vi "BCG Lookup.vi"() -> ()   [LabVIEW 2014]
doc: "This example shows how to apply a brightness, contrast, and gamma correction lookup table to an image. These transformations are usually applied to an image to improve its quality as required by a particular application."
uses:
  <vilib>/vision/NI_Vision_Development_Module.lvlib
panel:
  in  "Stop Button":bool
  out "Processed Image":T1(plugin-control)
  out "Image Source":T1(plugin-control)
  in  "BCG Values":T2={"Brightness"=171.0, "Contrast"=56.0, "Gamma"=2.0} {"Gamma" min=0.1 max=10 step=0.01 scale=10.0..0.1; "Contrast" min=1 max=89 step=1 scale=30.0..60.0; "Brightness" min=0 max=255 step=1 scale=0.0..255.0}
  # "Overview: Demonstrates how to improve the appearance of an image by changing brightness, contrast and gamma.\nRequirements: NI Vision Development Module\nInstructions: Run the VI."
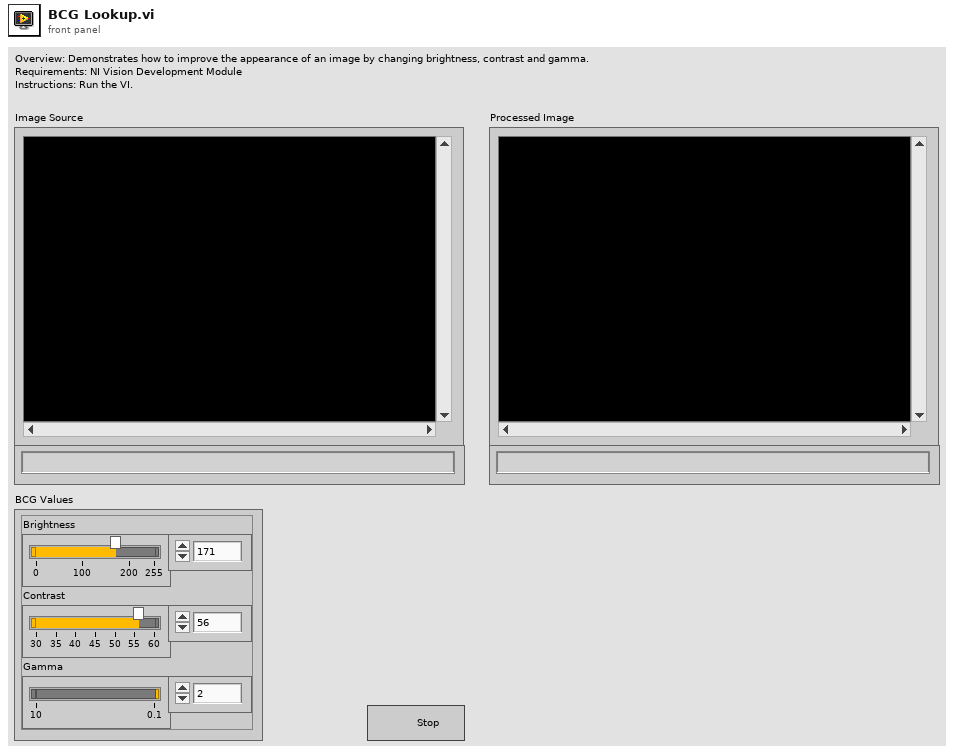
[diagram p1: front panel]
types:
  T1 = typedef "IMAQ Image.ctl" = refnum<image>
  T2 = cluster{"Brightness":sgl, "Contrast":sgl, "Gamma":sgl}
  T3 = typedef "Image Type" = u32
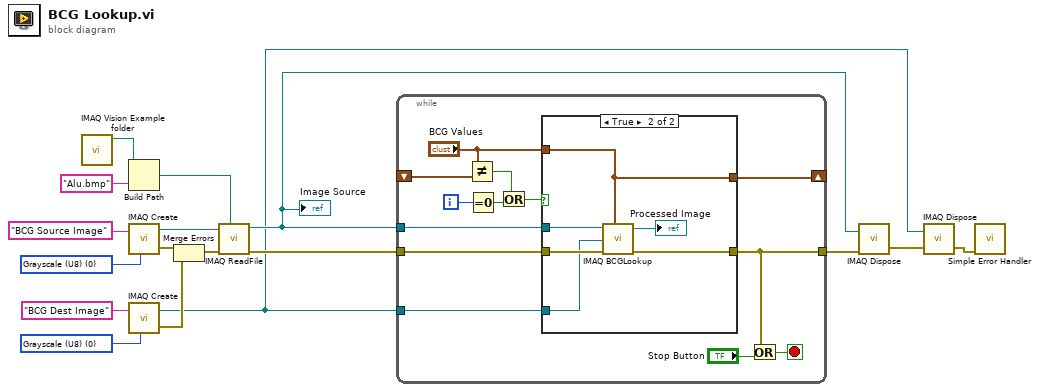
[diagram p0: block diagram]
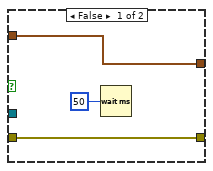
[diagram p2: hidden frame]
diagram:
  w8 = T3 0 items=["Grayscale (U8)", "Grayscale (I16)", "Grayscale (SGL)", "Complex (CSG)", "RGB (U32)", "HSL (U32)", "RGB (U64)", "Grayscale (U16)"] ("Image Type")
  w9 = T3 0 items=["Grayscale (U8)", "Grayscale (I16)", "Grayscale (SGL)", "Complex (CSG)", "RGB (U32)", "HSL (U32)", "RGB (U64)", "Grayscale (U16)"] ("Image Type")
  n1 = call "IMAQ Vision Example folder.vi"() -> ("Example Image Path"=w16:path)  [unwired: 11 in]
  n2 = Build Path(base path=w16, name or relative path="Alu.bmp") -> (appended path=w11:path)
  n3 = call "IMAQ Create"("Image Name"="BCG Source Image", "Image Type"=w9) -> ("New Image"=w12:T1, "error out"=w7:errorcluster)  [unwired: 3 in]
  n4 = call "IMAQ Create"("Image Name"="BCG Dest Image", "Image Type"=w8) -> ("New Image"=w1:T1, "error out"=w6:errorcluster)  [unwired: 3 in]
  n5 = Merge Errors(w7, w6) -> (w5:errorcluster)
  n6 = call "IMAQ ReadFile"("File Path"=w11, "error in (no error)"=w5, "Image"=w12) -> ("error out"=w10:errorcluster, "Image Out"=w2:T1)  [unwired: 4 in, 3 out]
  "Image Source" <- w2
  n7 = while {
    tunnel: w10 -> [w30]
    tunnel: w2 -> [w29]
    tunnel: w1 -> [w28]
    shift-right: [w27] -> _
    shift-left: _ -> [w26]
    tunnel: [w19] -> w17
    i -> [w24]
    stop <- w18 stop-if-true
    n8 = Not Equal?(x="BCG Values", y=w26) -> (x != y?=w23:bool)
    n9 = Equal To 0?(x=w24) -> (x = 0?=w22:bool)
    n10 = Or(x=w23, y=w22) -> (x .or. y?=w21:bool)
    n11 = case shown="True" w21 {
      tunnel: w30 -> [w33 w39]
      tunnel: w29 -> [_ w37]
      tunnel: "BCG Values" -> [w32 w35]
      tunnel: w28 -> [_ w36]
      tunnel: [w32 w35] -> w27
      tunnel: [w33 w34] -> w19
      frame False {
        n12 = Wait (ms)(milliseconds to wait=u32 50) -> ()  [unwired: 1 out]
      }
      frame True {
        n13 = call "IMAQ BCGLookup"("Image Src"=w37, "BCG Values"=w35, "Image Dst"=w36, "error in (no error)"=w39) -> ("Image Dst Out"=→"Processed Image":T1, "error out"=w34:errorcluster)  [unwired: 3 in]
      }
    }
    n14 = Or(x=w19, y="Stop Button") -> (x .or. y?=w18:bool)
  }
  n15 = call "IMAQ Dispose"("Image"=w2, "error in (no error)"=w17) -> ("error out"=w3:errorcluster)  [unwired: 4 in]
  n16 = call "IMAQ Dispose"("Image"=w1, "error in (no error)"=w3) -> ("error out"=w4:errorcluster)  [unwired: 4 in]
  n17 = call <vilib>:"Simple Error Handler.vi"("error in (no error)"=w4) -> ()  [unwired: 4 in, 5 out]
